vi "Shutdown Warning.vi"(11 "ConsoleView Sink in":refnum<class "ConsoleView.lvclass">) -> (2 "Shutdown?":bool, 3 "ConsoleView Sink Out":refnum<class "ConsoleView.lvclass">)   [LabVIEW 2020, in "ConsoleView.lvlib" / "ConsoleView.lvclass"]
uses:
  <vilib>/gpm_packages/@cs/event-logger/Source/ConsoleView/View/ConsoleView.lvclass
  <vilib>/gpm_packages/@cs/event-logger/Source/ConsoleView/View/ConsoleView.lvclass/ConsoleView.ctl
panel:
  in  "Cancel":bool
  in  "Hide and Disable":bool
  in  "Hide":bool
  in  "Shutdown":bool
  # "You have closed the console view window, however the console sink is still active, and the deferred shutdown option is marked true. How would you like to proceed?"
  # "Select if you are completely done with the console view"
  # "Select if you would like to hide the view, and shutdown when the logger stops."
  # "Select to hide the view. You must explicitly close the console session via the console API, or the view will continue to run after logger close."
  # "Cancel the close operation and return to the view."
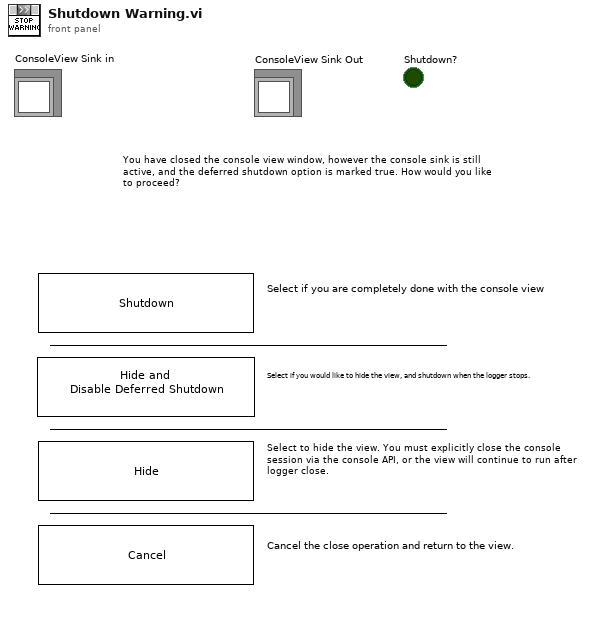
[diagram p1: front panel]
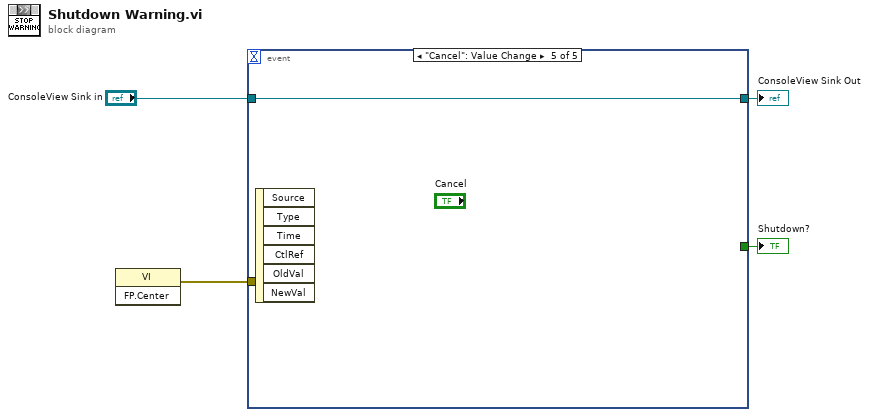
[diagram p0: block diagram]
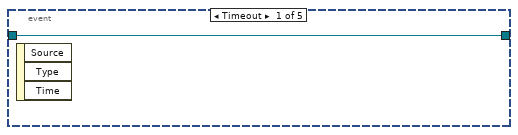
[diagram p2: hidden frame]
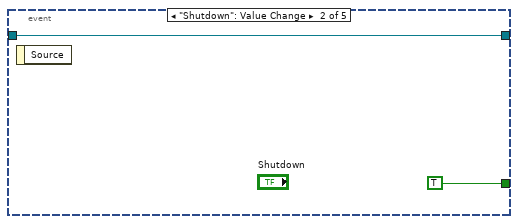
[diagram p3: hidden frame]
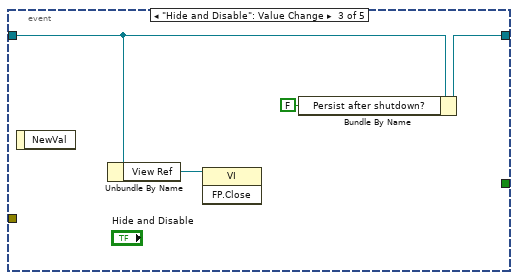
[diagram p4: hidden frame]
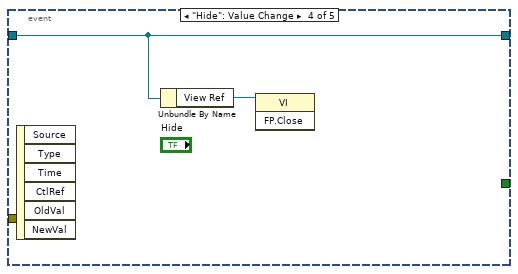
[diagram p5: hidden frame]
diagram:
  n1 = invoke class="VI" method="FP.Center"() -> (error out=w1:errorcluster)  [unwired: 3 in, 2 out]
  n2 = event shown="[4] \"Cancel\": Value Change" {
    selector: _ -> [_ _ _ _ _]
    dyn-events: _ -> [_ _ _ _ _]
    timeout: _ -> [_ _ _ _ _]
    tunnel: "ConsoleView Sink in" -> [w5 w7 w11 w12 w14]
    tunnel: [w5 w7 w9 w12 w14] -> w3
    tunnel: [_ TRUE _ _ _] -> w2
    tunnel: w1 -> [_ _ _ _ _]
    event Timeout {
      n3 = event-data() -> ()  [unwired: 1 in, 3 out]
    }
    event "Shutdown": Value Change {
      n4 = event-data() -> ()  [unwired: 1 in, 1 out]
    }
    event "Hide and Disable": Value Change {
      n5 = event-data() -> ()  [unwired: 1 in, 1 out]
      n6 = Unbundle By Name(w11) -> ("View Ref"=w10:refnum<vi>)
      n7 = invoke class="VI" method="FP.Close"(reference=w10) -> ()  [unwired: 2 in, 3 out]
      n8 = Bundle By Name(cluster=w11, "Persist after shutdown?"=FALSE) -> (w9:refnum<class "ConsoleView.lvclass">)
    }
    event "Hide": Value Change {
      n9 = event-data() -> ()  [unwired: 1 in, 6 out]
      n10 = Unbundle By Name(w12) -> ("View Ref"=w13:refnum<vi>)
      n11 = invoke class="VI" method="FP.Close"(reference=w13) -> ()  [unwired: 2 in, 3 out]
    }
    event "Cancel": Value Change {
      n12 = event-data() -> ()  [unwired: 1 in, 6 out]
    }
  }
  "ConsoleView Sink Out" <- w3
  "Shutdown?" <- w2
